vi "State.vi"() -> (3 "state":dbl[](array[numeric]))   [LabVIEW 2017]
uses:
  Global.vi
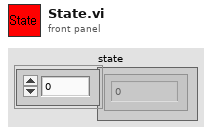
[diagram p1: front panel]
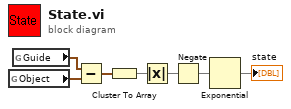
[diagram p0: block diagram]
diagram:
  n1 = global read "Global.vi" "Object"() -> (w1:cluster{"roll":dbl, "pitch":dbl, "yaw":dbl})
  n2 = global read "Global.vi" "Guide"() -> (w2:cluster{"roll":dbl, "pitch":dbl, "yaw":dbl})
  n3 = Subtract(x=w2, y=w1) -> (x-y=w3:cluster{"roll":dbl, "pitch":dbl, "yaw":dbl})
  n4 = Cluster To Array(cluster=w3) -> (array=w6:dbl[])
  n5 = Absolute Value(x=w6) -> (abs(x)=w7:dbl[])
  n6 = Negate(x=w7) -> (-x=w4:dbl[])
  n7 = Exponential(1:w4) -> (0:→"state":dbl[])
